vi "Launch Topic.vi"(7 "Include Initial Value? (F)":bool, 9 "Type":variant, 10 "Datum Name":string, 11 "Mediator in":refnum<class "Mediator.lvclass">) -> (0 "error out":errorcluster, 2 "New Topic Enqueuer":refnum<class "Message Enqueuer.lvclass">, 3 "Mediator out":refnum<class "Mediator.lvclass">)   [LabVIEW 2020, in "Mediator.lvlib" / "Mediator.lvclass"]
uses:
  <vilib>/gpm_packages/@cs/mva-core/Source/Mediator/Mediator/Mediator.lvclass
  C:/Program Files/National Instruments/LabVIEW 2020/vi.lib/ActorFramework/Actor/Actor.lvclass
  C:/Program Files/National Instruments/LabVIEW 2020/vi.lib/gpm_packages/@cs/mva-core/Source/IMediator/IMediator/IMediator.lvclass
  <vilib>/ActorFramework/Message Enqueuer/Message Enqueuer.lvclass
  <vilib>/gpm_packages/@cs/mva-core/Source/IMediator/IMediator/IMediator.lvclass/IMediator.ctl
  <vilib>/gpm_packages/@cs/mva-core/Source/Mediator/Topic/Topic.lvclass/Topic.ctl
  <vilib>/gpm_packages/@cs/mva-core/Source/Mediator/Mediator/Mediator.lvclass/Mediator.ctl
  <vilib>/gpm_packages/@cs/mva-core/Source/Mediator/TopicLookupTable/TopicLookupTable.lvclass/TopicLookupTable.ctl
  <vilib>/gpm_packages/@cs/mva-core/Source/Mediator/Topic/Read Topic Info.vi
  <vilib>/ActorFramework/Actor/Read Self Enqueuer.vi
  <vilib>/ActorFramework/Message Enqueuer/Init from Existing Queue.vi
  <vilib>/gpm_packages/@cs/mva-core/Source/Mediator/Topic/Topic.lvclass
  <vilib>/gpm_packages/@cs/variant/Source/Format Type String.vi
  <vilib>/ErrorRing/Error Ring.xnode
  <vilib>/ActorFramework/Actor/Actor.lvclass
  <vilib>/gpm_packages/@cs/mva-core/Source/Mediator/TopicLookupTable/TopicLookupTable.lvclass
  <vilib>/gpm_packages/@cs/mva-core/Source/IMediator/IMediator/IMediator.lvclass
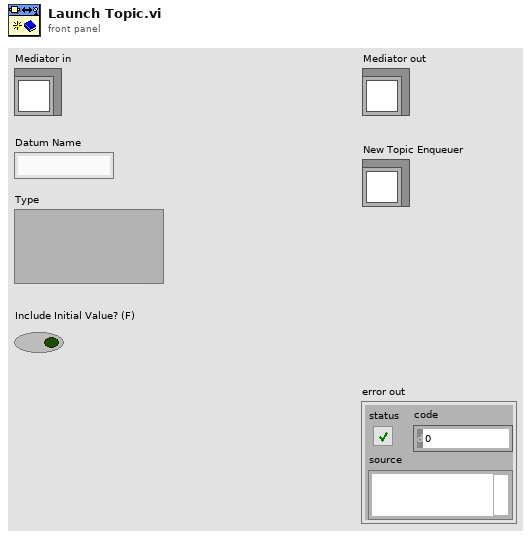
[diagram p1: front panel]
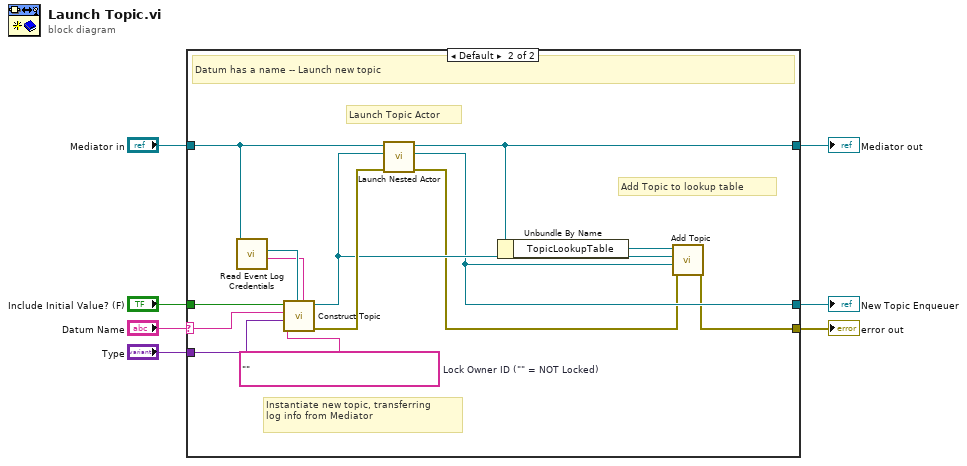
[diagram p0: block diagram]
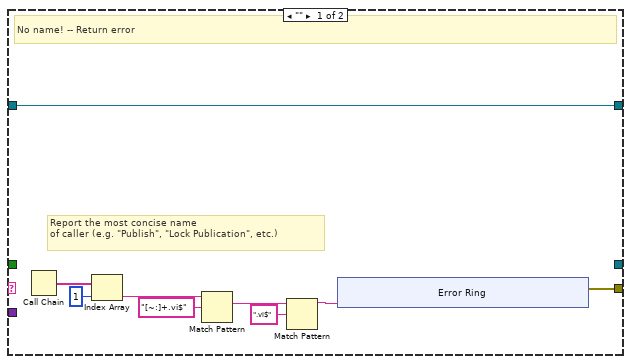
[diagram p2: hidden frame]
diagram:
  n1 = case shown="Default" "Datum Name" {
    selector: "Datum Name" -> [_ w29]
    tunnel: "Type" -> [_ w35]
    tunnel: [w16 w31] -> w2
    tunnel: "Include Initial Value? (F)" -> [_ w30]
    tunnel: "Mediator in" -> [w16 w27]
    tunnel: [_ w24] -> w3
    tunnel: [w15 w22] -> w1
    frame "" {
      # "Report the most concise name\nof caller (e.g. \"Publish\", \"Lock Publication\", etc.)"
      # "No name! -- Return error"
      n2 = Call Chain() -> (call chain=w14:string[])
      n3 = Index Array(array=w14, index=1) -> (element=w12:string)
      n4 = Match Pattern(string=w12, regular expression="[~:]+.vi$") -> (match substring=w11:string)  [unwired: 1 in, 3 out]
      n5 = Match Pattern(string=w11, regular expression=".vi$") -> (before substring=w9:string)  [unwired: 1 in, 3 out]
      n6 = xnode "Error Ring"("parameter 0"=w9) -> ("error out"=w15:errorcluster)
    }
    frame Default {
      w28 = ""  # Lock Owner ID ("" = NOT Locked)
      # "Launch Topic Actor"
      # "Add Topic to lookup table"
      # "Instantiate new topic, transferring\nlog info from Mediator"
      # "Datum has a name -- Launch new topic"
      n7 = call <vilib>:"Read Event Log Credentials.vi"("IMediator in"=w27) -> ("Framework Instance Alias"=w25:string, "Event Log Instance"=w26:refnum<class "LoggerReference.lvclass">)  [unwired: 9 in]
      n8 = call <vilib>:"Construct Topic.vi"("Framework Instance Alias"=w25, "Event Log Instance"=w26, "Lock Owner ID (\"\" = NOT Locked)"=w28, "New Topic Data"=w35, "Name"=w29, "Use Type Input As Initial Value?"=w30) -> ("error out"=w34:errorcluster, "Topic out"=w33:refnum<class "Topic.lvclass">)  [unwired: 4 in]
      n9 = call <vilib>:"Launch Nested Actor.vi"("error in (no error)"=w34, "Nested Actor"=w33, "Caller Actor in"=w27) -> ("error out"=w23:errorcluster, "Nested Actor's Enqueuer"=w24:refnum<class "Message Enqueuer.lvclass">, "Caller Actor out"=w31:refnum<class "Mediator.lvclass">)  [unwired: 6 in]
      n10 = Unbundle By Name(w31) -> ("TopicLookupTable"=w32:refnum<data-value>)
      n11 = call <vilib>:"Add Topic.vi"("error in (no error)"=w23, "Topic Enqueuer"=w24, "Topic Object"=w33, "TopicLookupTable"=w32) -> ("error out"=w22:errorcluster)  [unwired: 5 in, 2 out]
    }
  }
  "error out" <- w1
  "New Topic Enqueuer" <- w3
  "Mediator out" <- w2
